vi "new.vi"(6 "parameter":string, 8 "error in (no error)":errorcluster, 9 "function":string, 10 "id":string, 11 "result":refnum<class "result.lvclass">) -> (0 "error Out":errorcluster, 3 "result":refnum<class "result.lvclass">)   [LabVIEW 2015, in "result.lvclass"]
uses:
  result.lvclass
  result.lvclass/result.ctl
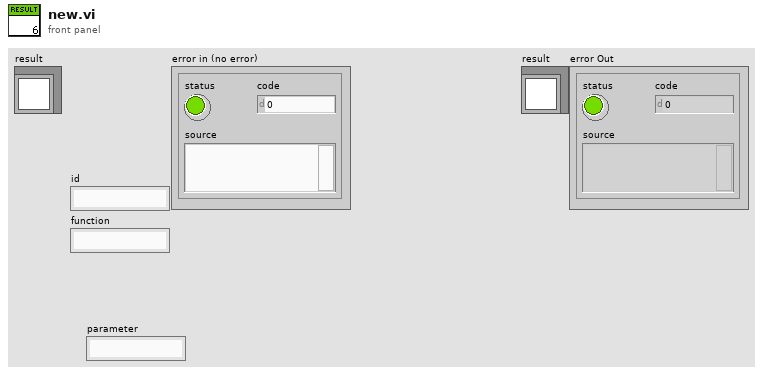
[diagram p1: front panel]
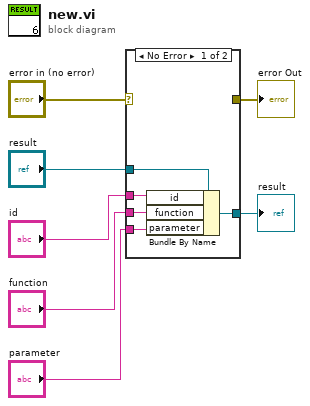
[diagram p0: block diagram]
diagram:
  n1 = case shown="No Error" "error in (no error)" {
    selector: "error in (no error)" -> [_ w13]
    tunnel: "id" -> [w12 _]
    tunnel: "function" -> [w11 _]
    tunnel: [w10 _] -> w5
    tunnel: "parameter" -> [w9 _]
    tunnel: [_ w13] -> w2
    tunnel: "result" -> [w8 _]
    frame No Error {
      n2 = Bundle By Name(cluster=w8, "id"=w12, "function"=w11, "parameter"=w9) -> (w10:refnum<class "result.lvclass">)
    }
    frame Error {
    }
  }
  "result" <- w5
  "error Out" <- w2
